vi "PH_Interaction.Save MCL Listbox Data to Harddisk.vi"(0 "VI in":refnum<vi>, 2 "Headline":string, 3 "MCL Listbox GUI Reference":refnum<vi>, 5 "error in (no error)":errorcluster) -> (14 "VI out":refnum<vi>, 19 "error out":errorcluster)   [LabVIEW 2014, in "PH_Common.lvlib"]
doc: "This VI is forseen to save MCL Listbox Data to harddisk."
uses:
  PH_Common.lvlib
  Names/PH_Names.File Types.ctl
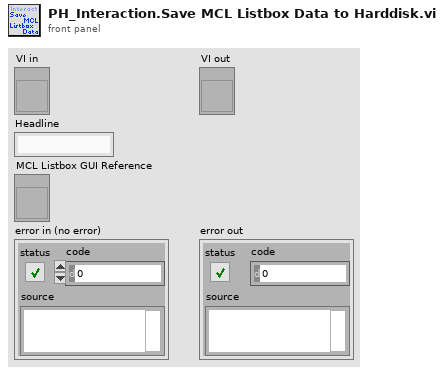
[diagram p1: front panel]
types:
  T1 = typedef "PH_Common.lvlib/PH_Names.File Types.ctl" = string
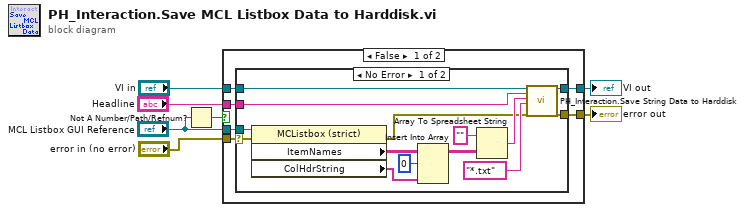
[diagram p0: block diagram]
diagram:
  n1 = Not A Number/Path/Refnum?(number/path/refnum="MCL Listbox GUI Reference") -> (NaN/Path/Refnum?=w2:bool)
  n2 = case shown="False" w2 {
    tunnel: "Headline" -> [w13 _]
    tunnel: [w12 w31] -> w6
    tunnel: "VI in" -> [w11 w31]
    tunnel: [w10 w30] -> w4
    tunnel: "error in (no error)" -> [w8 w30]
    tunnel: "MCL Listbox GUI Reference" -> [w9 _]
    frame False {
      n3 = case shown="No Error" w8 {
        selector: w8 -> [w14 w28]
        tunnel: w13 -> [w25 _]
        tunnel: [w24 w29] -> w12
        tunnel: w11 -> [w23 w29]
        tunnel: [w22 w28] -> w10
        tunnel: w9 -> [w15 _]
        frame No Error {
          n4 = property class="MCListbox (strict)"(reference=w15, error in=w14) -> (error out=w17:errorcluster, "ItemNames"=w19:string[][], "ColHdrString"=w18:string[])  [unwired: 1 out]
          n5 = Insert Into Array(array=w19, index (row)=0, new element=w18) -> (w16:string[][])  [unwired: 1 in]
          n6 = Array To Spreadsheet String(array=w16, 3:"" ("format string")) -> (spreadsheet string=w26:string)  [unwired: 1 in]
          n7 = call "PH_Interaction.Save String Data to Harddisk.vi"("i ref in"=w23, "Explanation (for Example: Column 1: xxx, ...)"=w25, "Data (for example: Columns)"=w26, "file name extension"=T1 "*.txt", "error in (no error)"=w17) -> ("i ref out"=w24:refnum<vi>, "error out"=w22:errorcluster)  [unwired: 12 in, 1 out]
        }
        frame Error {
        }
      }
    }
    frame True {
    }
  }
  "VI out" <- w6
  "error out" <- w4
